vi "DAC dp PD23X FP Conf.vi"(8 "error in (no error)":errorcluster, 9 "Used dp PD23X":bool[](array[boolean]), 10 "Result Unit":string, 11 "DeepU Results in":refnum<class "DeepU Results.lvclass">) -> (0 "error out":errorcluster, 3 "DeepU Results out":refnum<class "DeepU Results.lvclass">)   [LabVIEW 2019, in "Results.lvlib" / "DeepU Results.lvclass"]
uses:
  DeepU Results.lvclass
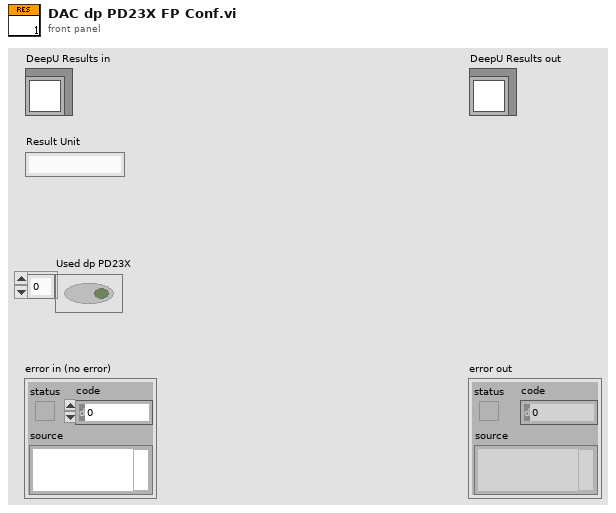
[diagram p1: front panel]
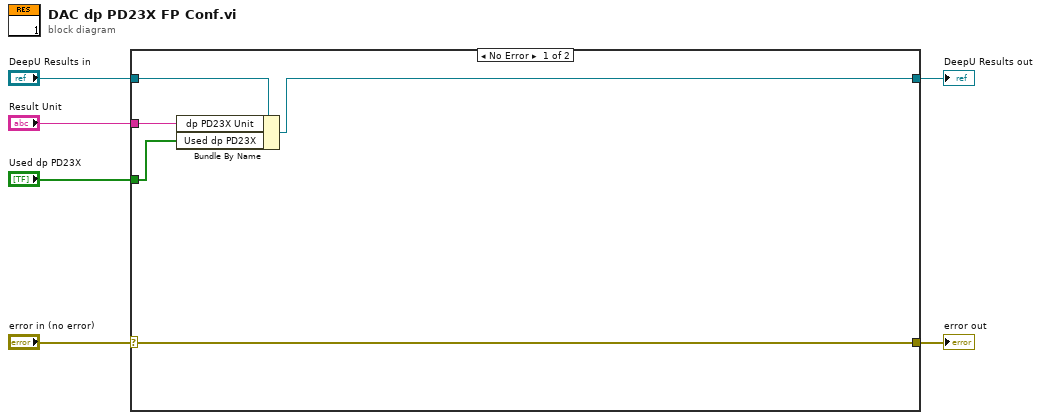
[diagram p0: block diagram]
diagram:
  n1 = case shown="No Error" "error in (no error)" {
    selector: "error in (no error)" -> [w11 w13]
    tunnel: [w11 w13] -> w5
    tunnel: [w10 w12] -> w3
    tunnel: "DeepU Results in" -> [w9 w12]
    tunnel: "Result Unit" -> [w8 _]
    tunnel: "Used dp PD23X" -> [w7 _]
    frame No Error {
      n2 = Bundle By Name(cluster=w9, "dp PD23X Unit"=w8, "Used dp PD23X"=w7) -> (w10:refnum<class "DeepU Results.lvclass">)
    }
    frame Error {
    }
  }
  "error out" <- w5
  "DeepU Results out" <- w3
